vi "Dispense FN - OFF (SubVI).vi"(0 "Signals IN":T2={"Dispense"=FALSE, "Fill"=FALSE, "Spray"=FALSE, "Drain"=TRUE, "Complete"=FALSE, "Fill Error"=FALSE, "Dispense Error"=FALSE, "Fill Timeout"=FALSE, "Dispense Timeout"=FALSE}, 1 "Values IN":T3 {"Time Elapsed (s)" format="%.2f"; "Time Target (s)" format="%.2f"; "Dynamic Setpoint (g)" format="%.2f"; "Static Setpoint (g)" format="%.2f"; "Grams to Setpoint" format="%.2f"; "Adjusted Mass (g)" format="%.2f"; "Dispense Rate (g/sec)" format="%.2f"; "Fill Mass (g)" format="%.2f"; "Fill Rate (g/sec)" format="%.2f"}, 2 "Settings":T1={"ON Settings"={"Enable Dynamic Setpoint?"=TRUE, "Enable Dynamic Dispense Time?"=TRUE, "Enable Drain Rate Functions"=TRUE, "Dispense Sample Time (s)"=0.5, "Dispense Slope Ave"=0, "ON Timeout (sec)"=600.0, "1st Setpoint (% of Target)"=0.0, "2nd Setpoint (% of Target)"=0.0, "3rd Setpoint (% of Target)"=0.0, "Measure Dispense Delay (sec)"=0.0, "Settle Slope Sample Time (s)"=0.0}, "OFF Settings"={"Drain Sample Time (s)"=0.5, "Drain Rate Ave Size"=5, "Drain Rate Limits (± g/sec)"=10.0, "Level Slope Range (± g/sec)"=0.25, "OFF Timeout (sec)"=0.0, "Near SP Slope Level (± g/sec)"=0.01, "Near Setpoint Threshold (%)"=95.0}, "Overshoot Settings"={"Time Limit (s)"=60.0, "Container MAX (g)"=1500.0, "Max FILL Slope (+/- g/sec)"=10.0, "% Overshot to Enable (>)"=0.25}, "FILL Timeout (s)"=300.0, "Full Settle Time (s)"=3.0, "Pre-Hydrate \nSpray Time (s)"=10.0, "Pre-Hydrate \nWait Time (s)"=30.0}, 3 "Measured Mass (g)":dbl, 5 "State Change?":bool) -> (14 "Signals OUT":T2={"Dispense"=FALSE, "Fill"=FALSE, "Spray"=FALSE, "Drain"=TRUE, "Complete"=FALSE, "Fill Error"=FALSE, "Dispense Error"=FALSE, "Fill Timeout"=FALSE, "Dispense Timeout"=FALSE}, 15 "Values OUT":T3 {"Time Elapsed (s)" format="%.2f"; "Time Target (s)" format="%.2f"; "Dynamic Setpoint (g)" format="%.2f"; "Static Setpoint (g)" format="%.2f"; "Grams to Setpoint" format="%.2f"; "Adjusted Mass (g)" format="%.2f"; "Dispense Rate (g/sec)" format="%.2f"; "Fill Mass (g)" format="%.2f"; "Fill Rate (g/sec)" format="%.2f"}, 19 "ON Signal":bool)   [LabVIEW 2009]
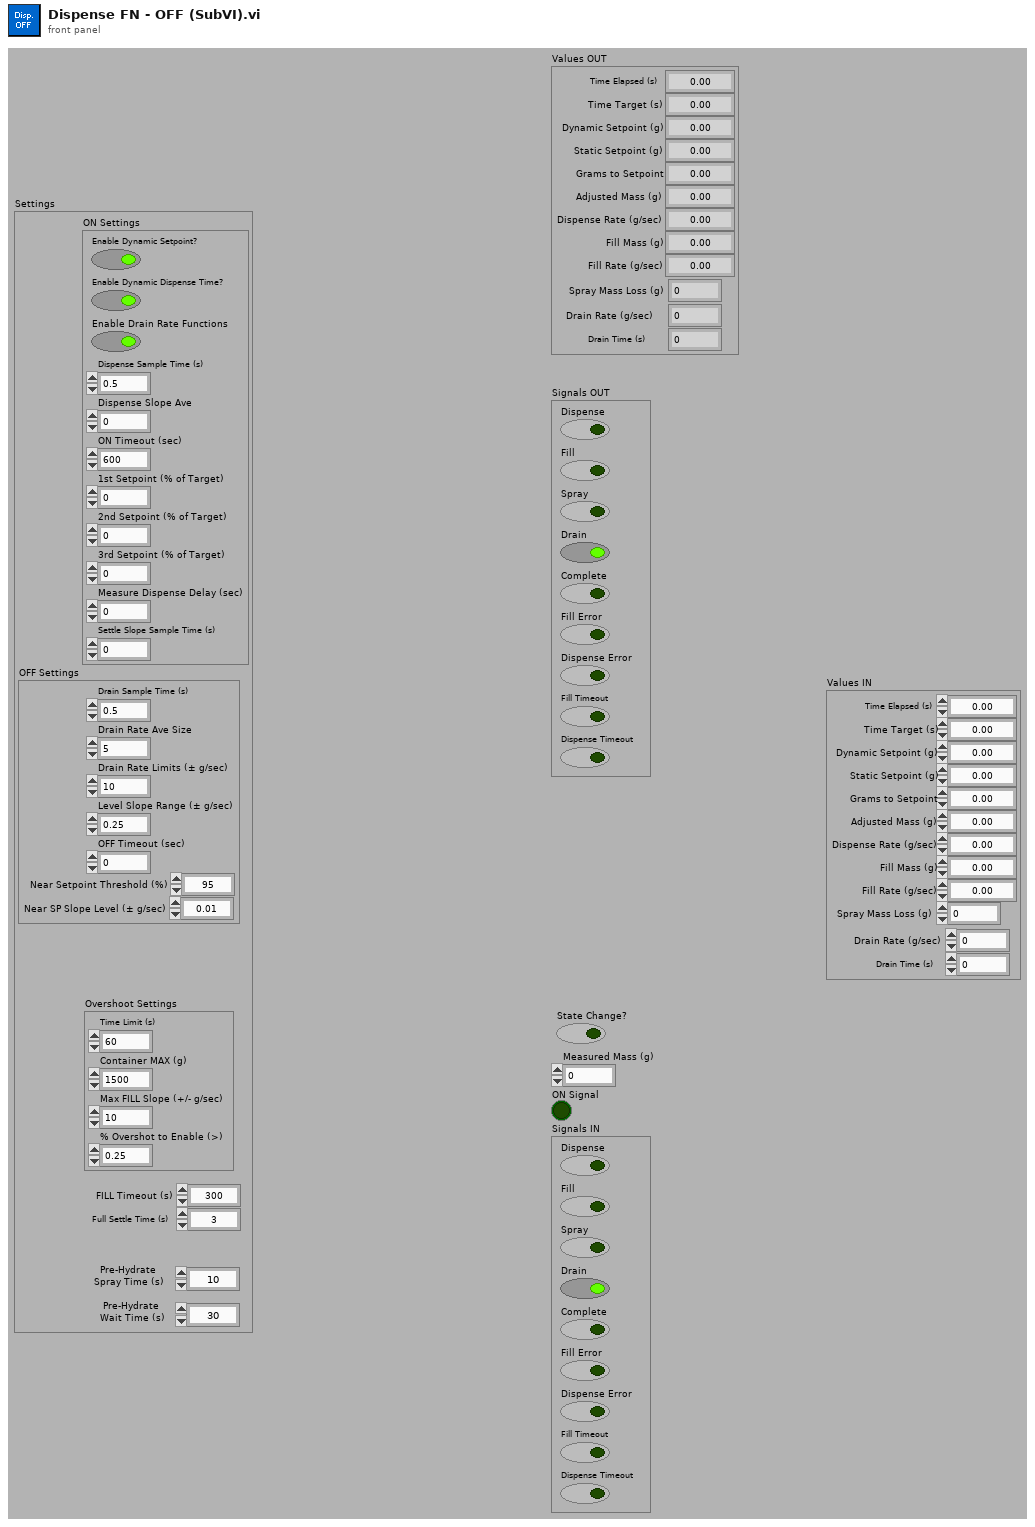
[diagram p1: front panel]
types:
  T1 = cluster{"ON Settings":cluster{"Enable Dynamic Setpoint?":bool, "Enable Dynamic Dispense Time?":bool, "Enable Drain Rate Functions":bool, "Dispense Sample Time (s)":dbl, "Dispense Slope Ave":i32, "ON Timeout (sec)":dbl, "1st Setpoint (% of Target)":dbl, "2nd Setpoint (% of Target)":dbl, "3rd Setpoint (% of Target)":dbl, "Measure Dispense Delay (sec)":dbl, "Settle Slope Sample Time (s)":dbl}, "OFF Settings":cluster{"Drain Sample Time (s)":dbl, "Drain Rate Ave Size":i32, "Drain Rate Limits (± g/sec)":dbl, "Level Slope Range (± g/sec)":dbl, "OFF Timeout (sec)":dbl, "Near SP Slope Level (± g/sec)":dbl, "Near Setpoint Threshold (%)":dbl}, "Overshoot Settings":cluster{"Time Limit (s)":dbl, "Container MAX (g)":dbl, "Max FILL Slope (+/- g/sec)":dbl, "% Overshot to Enable (>)":dbl}, "FILL Timeout (s)":dbl, "Full Settle Time (s)":dbl, "Pre-Hydrate \nSpray Time (s)":dbl, "Pre-Hydrate \nWait Time (s)":dbl}
  T2 = cluster{"Dispense":bool, "Fill":bool, "Spray":bool, "Drain":bool, "Complete":bool, "Fill Error":bool, "Dispense Error":bool, "Fill Timeout":bool, "Dispense Timeout":bool}
  T3 = cluster{"Time Elapsed (s)":dbl, "Time Target (s)":dbl, "Dynamic Setpoint (g)":dbl, "Static Setpoint (g)":dbl, "Grams to Setpoint":dbl, "Adjusted Mass (g)":dbl, "Dispense Rate (g/sec)":dbl, "Fill Mass (g)":dbl, "Fill Rate (g/sec)":dbl, "Spray Mass Loss (g)":dbl, "Drain Rate (g/sec)":dbl, "Drain Time (s)":dbl}
  T4 = cluster{"Settled Slope UL":dbl, "Settled Slope LL":dbl, "OFF Timeout (sec)":dbl, "Settle Slope Ave":i32, "Dispense Slope Ave":i32, "ON Timeout (sec)":dbl, "Dispense Slope Sample Time (s)":dbl, "1st Setpoint (% of Target)":dbl, "2nd Setpoint (% of Target)":dbl, "3rd Setpoint (% of Target)":dbl, "Enable Dynamic Setpoint?":bool, "Enable Dynamic Dispense Time?":bool, "Measure Dispense Delay (sec)":dbl, "Settle Slope Sample Time (s)":dbl}
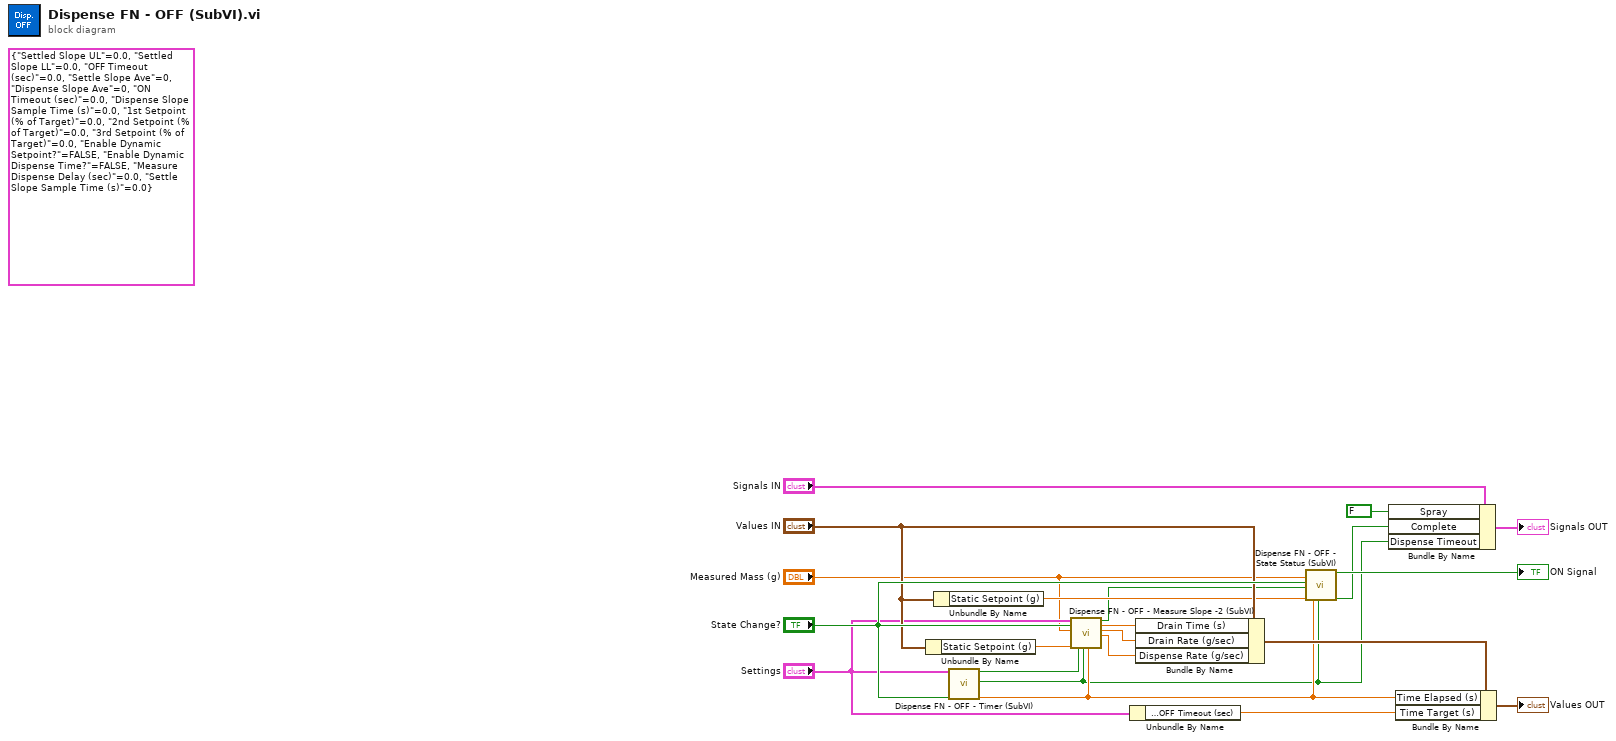
[diagram p0: block diagram]
diagram:
  (unwired) T4 {"Settled Slope UL"=0.0, "Settled Slope LL"=0.0, "OFF Timeout (sec)"=0.0, "Settle Slope Ave"=0, "Dispense Slope Ave"=0, "ON Timeout (sec)"=0.0, "Dispense Slope Sample Time (s)"=0.0, "1st Setpoint (% of Target)"=0.0, "2nd Setpoint (% of Target)"=0.0, "3rd Setpoint (% of Target)"=0.0, "Enable Dynamic Setpoint?"=FALSE, "Enable Dynamic Dispense Time?"=FALSE, "Measure Dispense Delay (sec)"=0.0, "Settle Slope Sample Time (s)"=0.0} ("Settings 2")
  n1 = Unbundle By Name("Values IN") -> ("Static Setpoint (g)"=w15:dbl)
  n2 = Unbundle By Name("Values IN") -> ("Static Setpoint (g)"=w11:dbl)
  n3 = call "Dispense FN - OFF - Timer (SubVI).vi"("Settings 2"="Settings", "Reset"="State Change?") -> ("Sample"=w16:bool, "Max Drain Complete?"=w1:bool, "Elapsed Time (s)"=w3:dbl)  [unwired: 15 in]
  n4 = call "Dispense FN - OFF - Measure Slope -2 (SubVI).vi"("Settings"="Settings", "Initialize"="State Change?", "Measured Mass (g)"="Measured Mass (g)", "Static Setpoint (g)"=w15, "Sample?"=w16, "Max Drain Complete?"=w1, "Elapsed Time (s)"=w3) -> ("Level Signal"=w10:bool, "Drain Time (s)"=w9:dbl, "Drain Rate (g/sec)"=w8:dbl, "Ave. Slope (g/sec)"=w7:dbl)  [unwired: 2 in, 7 out]
  n5 = Unbundle By Name("Settings") -> ("OFF Settings.OFF Timeout (sec)"=w4:dbl)
  n6 = Bundle By Name(cluster="Values IN", "Drain Time (s)"=w9, "Drain Rate (g/sec)"=w8, "Dispense Rate (g/sec)"=w7) -> (w17:T3)
  n7 = call "Dispense FN - OFF - State Status (SubVI).vi"("Measured Mass (g)"="Measured Mass (g)", "State Change Pulse"="State Change?", "Level Slope?"=w10, "Static Setpoint (g)"=w11, "Elapsed Time (s)"=w3, "Max Drain Complete?"=w1) -> ("ON Signal"=→"ON Signal":bool, "Complete"=w6:bool)  [unwired: 1 in, 11 out]
  n8 = Bundle By Name(cluster="Signals IN", "Spray"=FALSE, "Complete"=w6, "Dispense Timeout"=w1) -> (→"Signals OUT":T2)
  n9 = Bundle By Name(cluster=w17, "Time Elapsed (s)"=w3, "Time Target (s)"=w4) -> (→"Values OUT":T3)
